vi "Get_CPU_Load.vi"(8 "error in (no error)":errorcluster) -> (0 "error out":errorcluster, 3 "Numeric":dbl)   [LabVIEW 2017]
uses:
  <vilib>/NI_Real-Time Target Support.lvlib
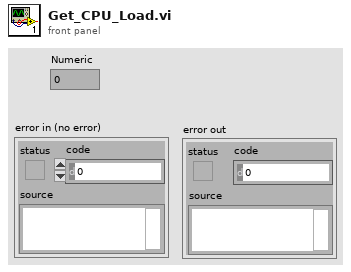
[diagram p1: front panel]
types:
  T1 = typedef "NI_Real-Time Target Support.lvlib/RT CPU Load.ctl" = cluster{"Total (%)":dbl, "Time Critical (%)":dbl, "Timed Structures (%)":dbl, "High (%)":dbl, "Above Normal (%)":dbl, "Normal (%)":dbl, "Background (%)":dbl, "Idle (%)":dbl, "ISR (%)":dbl}
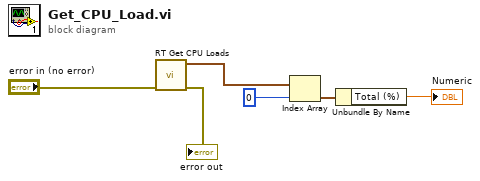
[diagram p0: block diagram]
diagram:
  n1 = call <vilib>:"RT Get CPU Loads.vi"("error in (no error)"="error in (no error)") -> ("error out"=→"error out":errorcluster, "CPU loads"=w3:T1[])  [unwired: 9 in]
  n2 = Index Array(array=w3, index=0) -> (element=w5:T1)
  n3 = Unbundle By Name(w5) -> ("Total (%)"=→"Numeric":dbl)
